vi "Generate_complex_sin.vi"(6 "Signal freq":dbl=0.2, 9 "SNR":dbl, 10 "Gain":dbl, 11 "Sampling Rate [Hz]":dbl) -> (3 "Waveform":waveform(cdb))   [LabVIEW 2018]
uses:
  <userlib>/_OpenG.lib/numeric/numeric.llb/Random Number Within Range - DBL__ogtk.vi
  <vilib>/measure/NI_MABase.lvlib
panel:
  out "Waveform Graph":dbl[][](graph)
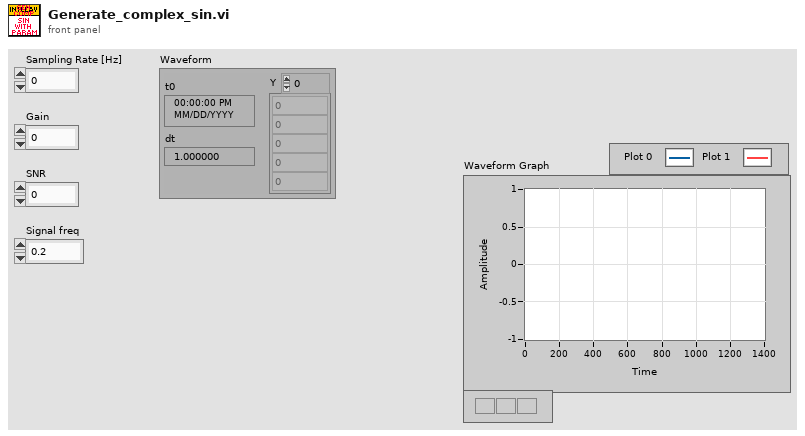
[diagram p1: front panel]
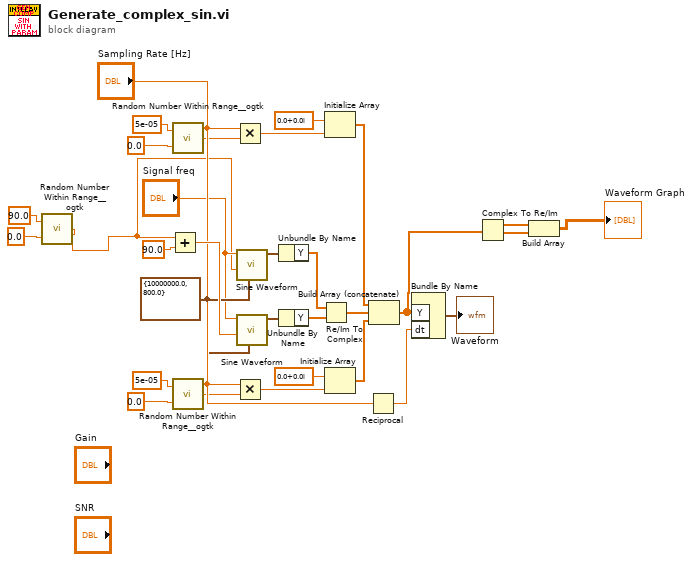
[diagram p0: block diagram]
diagram:
  w21 = cluster{"Fs":dbl, "#s":dbl} {"Fs"=10000000.0, "#s"=800.0} ("sampling info")
  n1 = call-poly <userlib>:"Random Number Within Range__ogtk.vi"("High"=90.0, "Low"=0.0) -> ("Random Number"=w1:dbl)  [unwired: 3 in]
  n2 = Add(x=w1, y=90.0 ("phase")) -> (x+y=w31:dbl)
  n3 = call-poly <userlib>:"Random Number Within Range__ogtk.vi"("High"=5e-05, "Low"=0.0) -> ("Random Number"=w24:dbl)  [unwired: 3 in]
  n4 = call-poly <userlib>:"Random Number Within Range__ogtk.vi"("High"=5e-05, "Low"=0.0) -> ("Random Number"=w26:dbl)  [unwired: 3 in]
  n5 = Multiply(x="Sampling Rate [Hz]", y=w24) -> (x*y=w8:dbl)
  n6 = Multiply(x="Sampling Rate [Hz]", y=w26) -> (x*y=w11:dbl)
  n7 = call <vilib>:"Sine Waveform.vi"("sampling info"=w21, "phase"=w1, "frequency"="Signal freq") -> ("signal out"=w16:waveform(dbl))  [unwired: 7 in, 1 out]
  n8 = call <vilib>:"Sine Waveform.vi"("sampling info"=w21, "phase"=w31, "frequency"="Signal freq") -> ("signal out"=w15:waveform(dbl))  [unwired: 7 in, 1 out]
  n9 = Unbundle By Name(w16) -> ("Y"=w19:dbl[])
  n10 = Unbundle By Name(w15) -> ("Y"=w20:dbl[])
  n11 = Re/Im To Complex(1:w20, 2:w19) -> (0:w17:cdb[])
  n12 = Initialize Array(cdb 0.0+0.0i ("element"), w8) -> (w9:cdb[])
  n13 = Initialize Array(cdb 0.0+0.0i ("element"), w11) -> (w12:cdb[])
  n14 = Reciprocal(x="Sampling Rate [Hz]") -> (1/x=w13:dbl)
  n15 = Build Array (concatenate)(w9, w17, w12) -> (w3:cdb[])
  n16 = Bundle By Name("Y"=w3, "dt"=w13) -> (→"Waveform":waveform(cdb))  [unwired: 1 in]
  n17 = Complex To Re/Im(x + iy=w3) -> (x=w6:dbl[], y=w5:dbl[])
  n18 = Build Array(w6, w5) -> (→"Waveform Graph":dbl[][])
